vi "Update Tree Control.vi"(10 "frame map":T2 {"value"."Type of Frame" items=["Raw Frame", "UDP/IP for Tx", "Tx UDP"]; "value"."Data" format="%.0x"}, 11 "Tree 2":refnum<vi>) -> ()   [LabVIEW 2020]
uses:
  <instrlib>/AIM GmbH/_AIM 664/AIM664LV.lvlib
  controls/Payload Record Type.ctl
  controls/Payload Map.ctl
  controls/Type of Payload.ctl
panel:
  in  "value.Type of Frame":T1 items=["Raw Frame", "UDP/IP for Tx", "Tx UDP"]
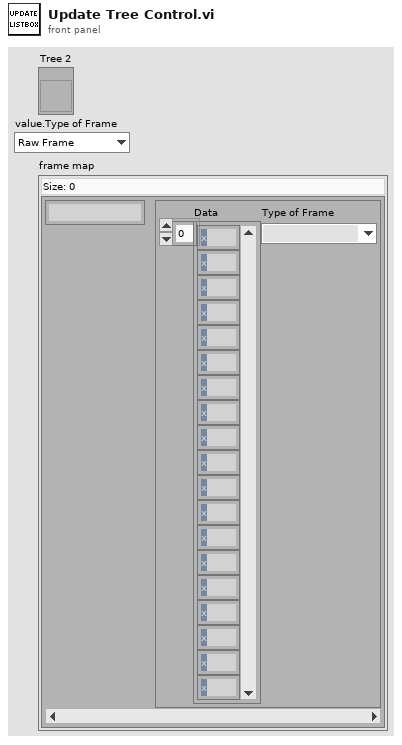
[diagram p1: front panel]
types:
  T1 = typedef "Type of Payload.ctl" = u16
  T2 = typedef "Payload Map.ctl" = map{string, T3}
  T3 = typedef "Payload Record Type.ctl" = cluster{"Data":u8[], "Type of Frame":T1}
  T4 = cluster{"Left Cell String":string, "Child Text":string[], "Child Tag":string, "Item Indent":i32, "Child Only?":bool, "Glyph Index":i32}
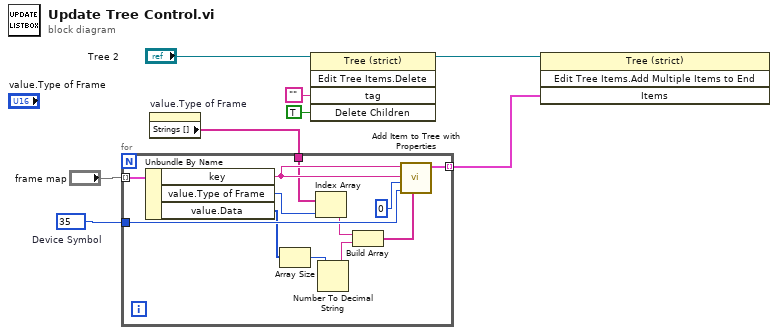
[diagram p0: block diagram]
diagram:
  w2 = 35  # Device Symbol
  n1 = property on="value.Type of Frame" class="Ring (strict)"() -> ("Strings []"=w1:string[])  [unwired: 2 in, 2 out]
  n2 = for {
    tunnel: "frame map" -> [w20] mode=indexing
    tunnel: [w18] -> w7 mode=indexing
    tunnel: w2 -> [w16]
    tunnel: w1 -> [w14]
    n3 = Unbundle By Name(w20) -> ("key"=w19:string, "value.Type of Frame"=w15:T1, "value.Data"=w11:u8[])
    n4 = Array Size(array=w11) -> (size(s)=w10:i32)
    n5 = Index Array(array=w14, index=w15) -> (element=w13:string)
    n6 = Number To Decimal String(number=w10) -> (decimal integer string=w9:string)  [unwired: 1 in]
    n7 = Build Array(w13, w9) -> (w12:string[])
    n8 = call <instrlib>:"Add Item to Tree with Properties.vi"("Child Text"=w12, "Glyph Index"=w16, "Item indent"=0, "Child Tag"=w19, "Left Cell String"=w19) -> ("Item"=w18:T4)  [unwired: 6 in]
  }
  n9 = invoke on="Invoke Node" class="Tree (strict)" method="Edit Tree Items.Delete"(reference="Tree 2", "tag"="", "Delete Children"=TRUE ("Delete Children?")) -> (reference out=w3:refnum<vi>)  [unwired: 2 in, 4 out]
  n10 = invoke on="Invoke Node" class="Tree (strict)" method="Edit Tree Items.Add Multiple Items to End"(reference=w3, "Items"=w7) -> ()  [unwired: 2 in, 4 out]
